vi "getSigProcessing.vi"(0 "Analogue Data (volts)":dbl[][](array[numeric])) -> (1 "Labelled Signals":string[][](array[string]), 2 "Channel Names":string[](array[string]), 3 "Raw Signals":dbl[][](array[numeric]))   [LabVIEW 2013]
uses:
  Globals/measurementGlobal.vi
panel:
  out "Chell Chans.":dbl[](array[numeric])
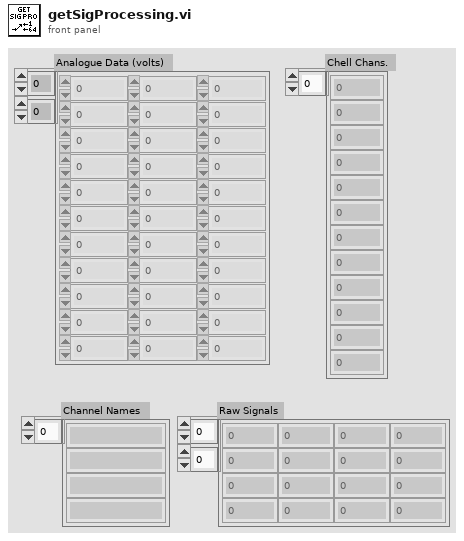
[diagram p1: front panel]
types:
  T1 = typedef "chanType.ctl" = enum16{"Default", "Clock", "Pressure Scanner"}
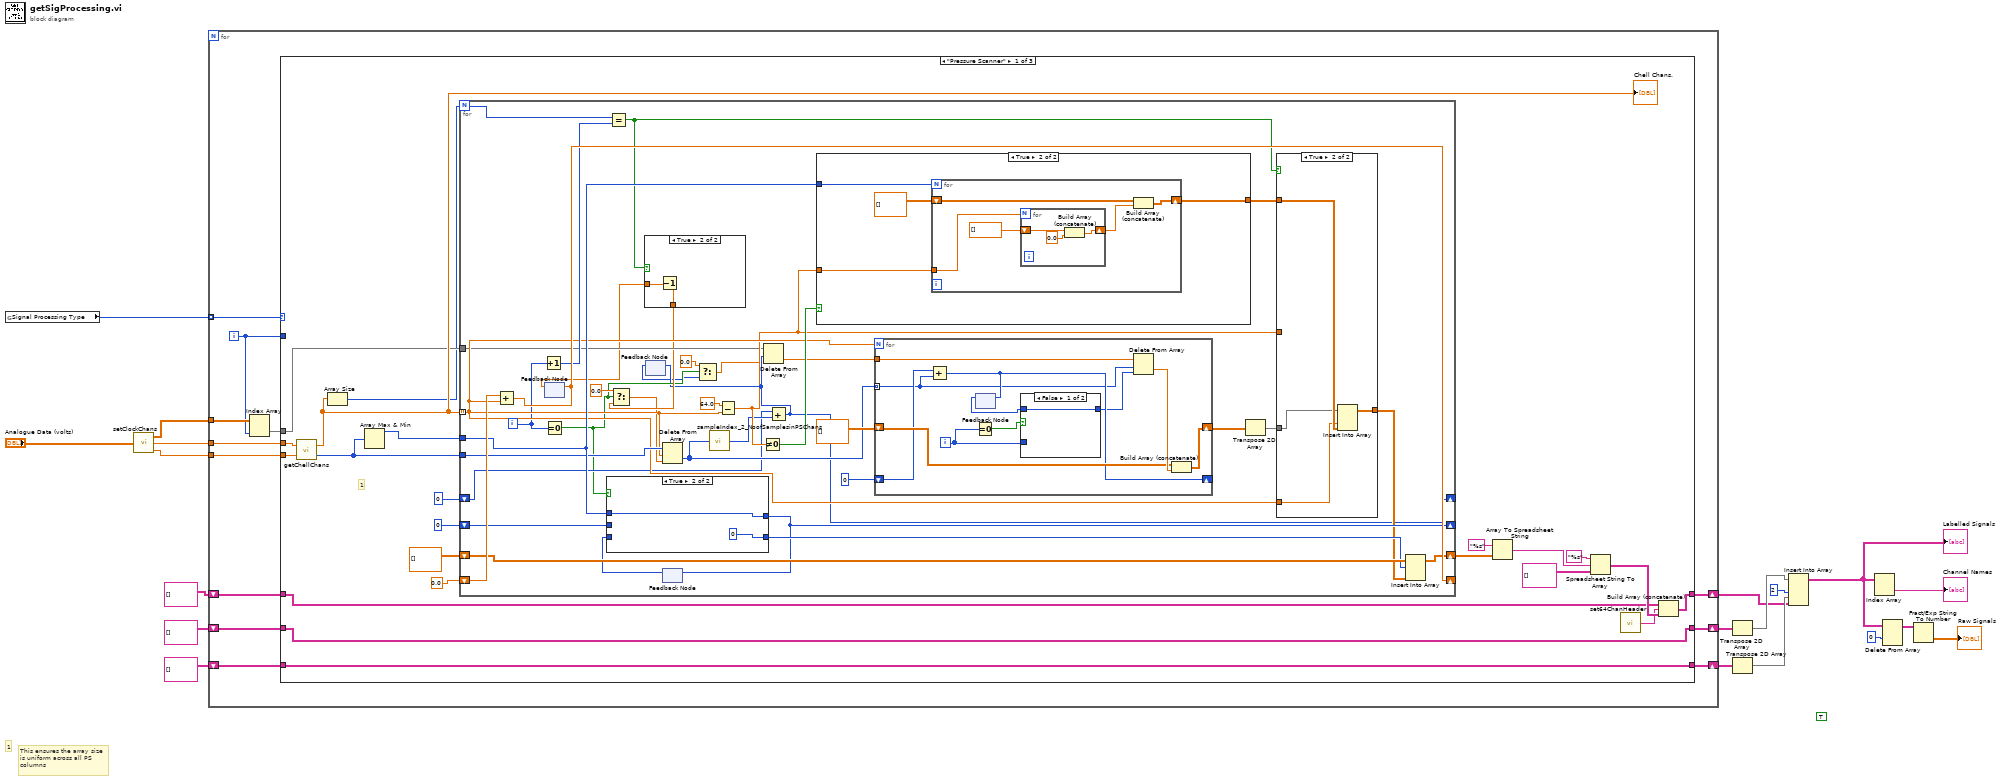
[diagram p0: block diagram]
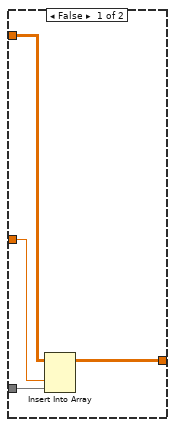
[diagram p3: hidden frame]
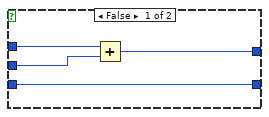
[diagram p4: hidden frame]
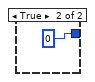
[diagram p5: hidden frame]
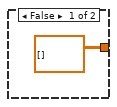
[diagram p6: hidden frame]
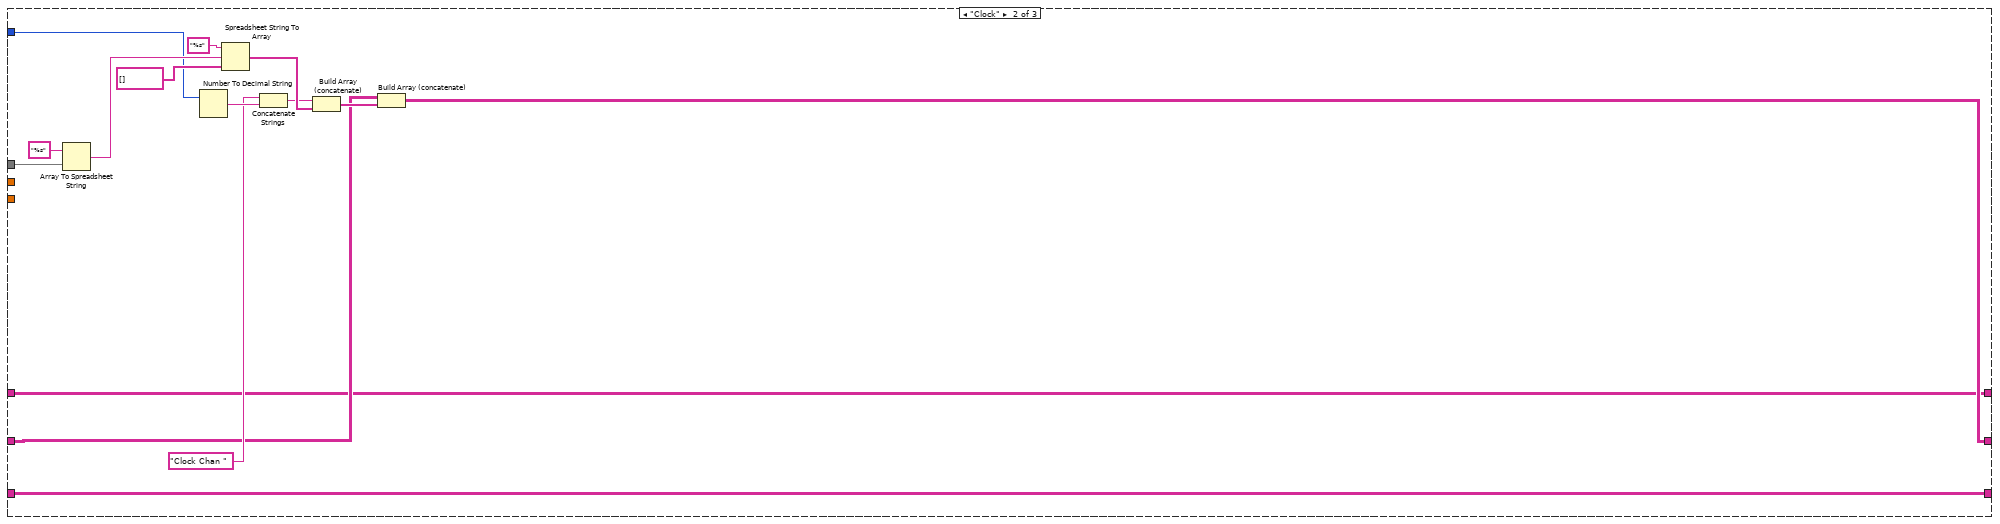
[diagram p7: hidden frame]
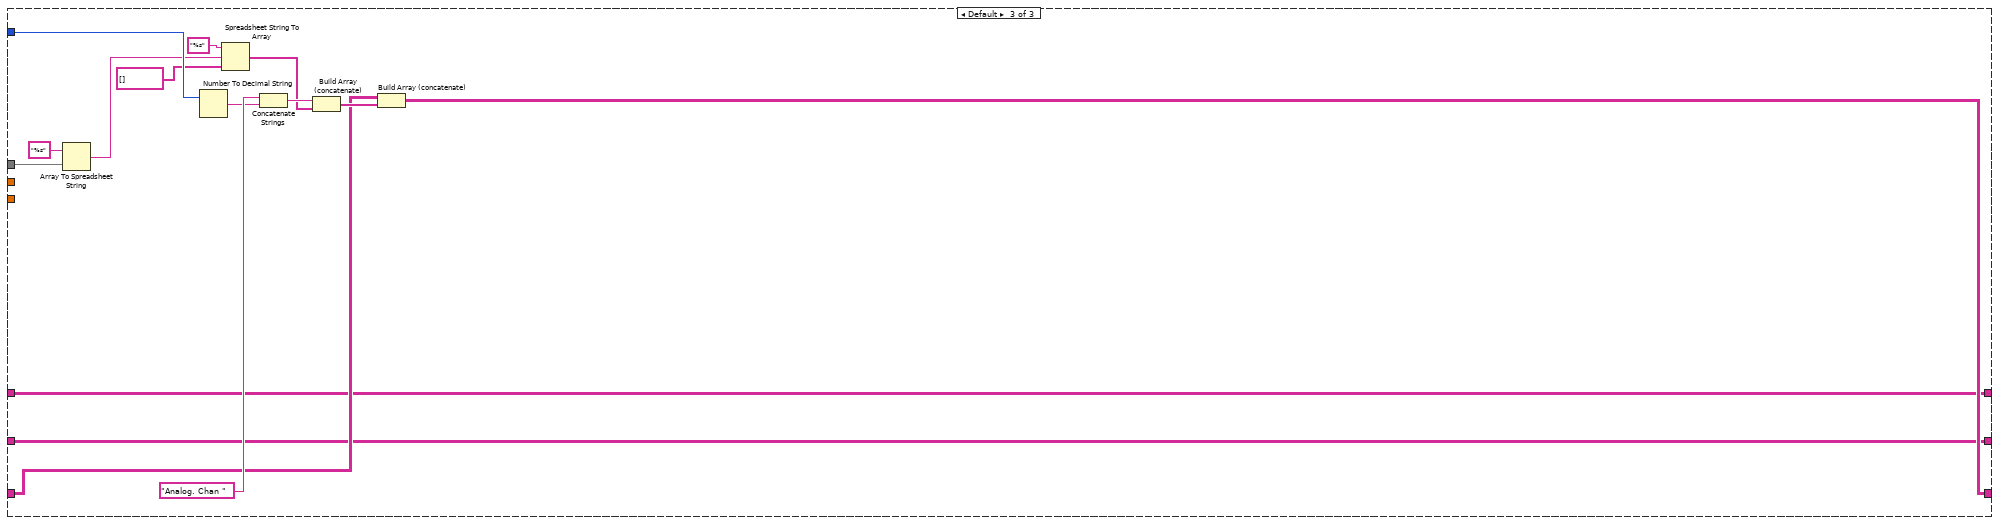
[diagram p8: hidden frame]
diagram:
  (unwired) TRUE
  # "1"
  # "This ensures the array size\nis uniform across all PS\ncolumns"
  n1 = global read "measurementGlobal.vi" "Signal Processing Type"() -> (w19:T1[])
  n2 = call "setClockChans.vi"("Analogue Data (volts)"="Analogue Data (volts)") -> ("Modified Analogue Data (volts)"=w12:dbl[][], "MSB"=w11:dbl[], "LSB"=w10:dbl[])
  n3 = for {
    tunnel: w19 -> [w20] mode=indexing
    tunnel: w12 -> [w30]
    tunnel: w11 -> [w29]
    tunnel: w10 -> [w28]
    shift-right: [w25] -> w7
    shift-left: string[][] [] -> [w26]
    shift-right: [w23] -> w3
    shift-left: string[][] [] -> [w24]
    shift-right: [w21] -> w1
    shift-left: string[][] [] -> [w22]
    i -> [w27]
    n4 = Index Array(array=w30, index (col)=w27) -> (element=w31:dbl[])  [unwired: 1 in]
    n5 = case shown="\"Pressure Scanner\"" w20 {
      tunnel: w31 -> [w45 w140 w150]
      tunnel: w29 -> [w53 _ _]
      tunnel: w28 -> [w52 _ _]
      tunnel: w27 -> [_ w141 w163]
      tunnel: w26 -> [w39 w138 w152]
      tunnel: [w39 w137 w152] -> w25
      tunnel: w24 -> [w38 w136 w154]
      tunnel: [w38 w136 w153] -> w23
      tunnel: w22 -> [w37 w135 w151]
      tunnel: [w36 w135 w151] -> w21
      frame "Pressure Scanner" {
        # "1"
        n6 = call "getChellChans.vi"("LSB"=w52, "MSB"=w53) -> ("Sample Index"=w51:i32[], "No. Chell Chans."=w48:dbl[])
        "Chell Chans." <- w48
        n7 = Array Size(array=w48) -> (size(s)=w33:i32)
        n8 = Array Max & Min(array=w51) -> (max value=w50:i32)  [unwired: 3 out]
        n9 = for {
          N: w33 -> [w77]
          tunnel: w48 -> [w74] mode=indexing
          tunnel: w45 -> [w69]
          tunnel: w51 -> [w79]
          tunnel: w50 -> [w84]
          shift-right: [w87] -> _
          shift-left: 0.0 -> [w88]
          shift-right: [w85] -> w35
          shift-left: dbl[][] [] ("array") -> [w86]
          shift-right: [w81] -> _
          shift-left: 0 -> [w82]
          shift-right: [w56] -> _
          shift-left: 0 -> [w59]
          i -> [w71]
          n10 = Add(x=w88, y=w74) -> (x+y=w87:dbl)
          n11 = Increment(x=w71) -> (x+1=w76:i32)
          n12 = feedback #1() -> (w64:dbl)  [unwired: 1 in]
          n13 = feedback-in #1(w87) -> ()
          n14 = Equal To 0?(x=w71) -> (x = 0?=w58:bool)
          n15 = Equal?(x=w77, y=w76) -> (x = y?=w65:bool)
          n16 = case shown="True" w65 {
            tunnel: w64 -> [w92 w94]
            tunnel: [w92 w93] -> w62
            frame False {
            }
            frame True {
              n17 = Decrement(x=w94) -> (x-1=w93:dbl)
            }
          }
          n18 = Select(t=0.0, s=w58, f=w62) -> (s? t:f=w61:dbl)
          n19 = feedback #2() -> (w55:i32)  [unwired: 1 in]
          n20 = Delete From Array(array=w79, length=w74, index=w61) -> (deleted portion=w66:i32[])  [unwired: 1 out]
          n21 = feedback #3() -> (w80:i32)  [unwired: 1 in]
          n22 = case shown="True" w58 {
            tunnel: w84 -> [w105 w108]
            tunnel: [w103 0] -> w83
            tunnel: w82 -> [w106 _]
            tunnel: [w104 w108] -> w81
            tunnel: w80 -> [w103 _]
            frame False {
              n23 = Add(x=w105, y=w106) -> (x+y=w104:i32)
            }
            frame True {
            }
          }
          n24 = feedback-in #3(w81) -> ()
          n25 = Select(t=0.0, s=w58, f=w55) -> (s? t:f=w54:dbl)
          n26 = call "sampleIndex_2_NoofSamplesinPSChans.vi"("Sample Index"=w66) -> ("No of Samples in PS Chans"=w60:i32)
          n27 = Subtract(x=64.0 ("y"), y=w74) -> (x-y=w73:dbl)
          n28 = Not Equal To 0?(x=w73) -> (x != 0?=w78:bool)
          n29 = Add(x=w59, y=w60) -> (x+y=w56:i32)
          n30 = feedback-in #2(w56) -> ()
          n31 = Delete From Array(array=w69, length=w56, index=w54) -> (deleted portion=w68:dbl[])  [unwired: 1 out]
          n32 = case shown="True" w78 {
            tunnel: w73 -> [_ w123]
            tunnel: [dbl[][] [] w126] -> w75
            tunnel: w84 -> [_ w125]
            frame False {
            }
            frame True {
              n33 = for {
                N: w125 -> [_]
                shift-right: [w128] -> w126
                shift-left: dbl[][] [] -> [w129]
                tunnel: w123 -> [w127]
                n34 = for {
                  N: w127 -> [_]
                  shift-right: [w133] -> w130
                  shift-left: dbl[] [] -> [w134]
                  n35 = Build Array (concatenate)(w134, 0.0) -> (w133:dbl[])
                }
                n36 = Build Array (concatenate)(w129, w130) -> (w128:dbl[][])
              }
            }
          }
          n37 = for {
            N: w74 -> [_]
            tunnel: w66 -> [w112] mode=indexing
            tunnel: w68 -> [w119]
            shift-right: [w117] -> w70
            shift-left: dbl[][] [] ("element") -> [w116]
            shift-right: [w114] -> _
            shift-left: 0 -> [w115]
            i -> [w111]
            n38 = Add(x=w115, y=w112) -> (x+y=w114:i32)
            n39 = feedback-in #4(w114) -> ()
            n40 = feedback #4() -> (w113:i32)  [unwired: 1 in]
            n41 = Equal To 0?(x=w111) -> (x = 0?=w110:bool)
            n42 = case shown="False" w110 {
              tunnel: [w120 0] -> w109
              tunnel: w111 -> [_ _]
              tunnel: w113 -> [w120 _]
              frame False {
              }
              frame True {
              }
            }
            n43 = Delete From Array(array=w119, length=w112, index=w109) -> (deleted portion=w118:dbl[])  [unwired: 1 out]
            n44 = Build Array (concatenate)(w116, w118) -> (w117:dbl[][])
          }
          n45 = Transpose 2D Array(2D array=w70) -> (transposed array=w67:dbl[][])
          n46 = case shown="True" w65 {
            tunnel: w75 -> [w98 w102]
            tunnel: w67 -> [w97 w101]
            tunnel: w74 -> [_ w99]
            tunnel: w73 -> [w96 _]
            tunnel: [w95 w100] -> w72
            frame False {
              n47 = Insert Into Array(array=w98, index (col)=w96, new element=w97) -> (w95:dbl[][])  [unwired: 1 in]
            }
            frame True {
              n48 = Insert Into Array(array=w101, index (col)=w99, new element=w102) -> (w100:dbl[][])  [unwired: 1 in]
            }
          }
          n49 = Insert Into Array(array=w86, index (row)=w83, new element=w72) -> (w85:dbl[][])  [unwired: 1 in]
        }
        n50 = Array To Spreadsheet String(array=w35, 3:"%s" ("format string")) -> (spreadsheet string=w43:string)  [unwired: 1 in]
        n51 = Spreadsheet String To Array(format string="%s", spreadsheet string=w43, array type (2D Dbl)=string[][] []) -> (array=w40:string[][])  [unwired: 1 in]
        n52 = call "set64ChanHeader.vi"() -> ("64 Chan Header"=w34:string[])
        n53 = Build Array (concatenate)(w37, w34, w40) -> (w36:string[][])
      }
      frame "Clock" {
        n54 = Array To Spreadsheet String(array=w140, 3:"%s" ("format string")) -> (spreadsheet string=w145:string)  [unwired: 1 in]
        n55 = Number To Decimal String(number=w141) -> (decimal integer string=w143:string)  [unwired: 1 in]
        n56 = Spreadsheet String To Array(format string="%s", spreadsheet string=w145, array type (2D Dbl)=string[] []) -> (array=w149:string[])  [unwired: 1 in]
        n57 = Concatenate Strings("Clock Chan " ("string"), w143) -> (w148:string)
        n58 = Build Array (concatenate)(w148, w149) -> (w139:string[])
        n59 = Build Array (concatenate)(w138, w139) -> (w137:string[][])
      }
      frame Default {
        n60 = Array To Spreadsheet String(array=w150, 3:"%s" ("format string")) -> (spreadsheet string=w160:string)  [unwired: 1 in]
        n61 = Number To Decimal String(number=w163) -> (decimal integer string=w162:string)  [unwired: 1 in]
        n62 = Spreadsheet String To Array(format string="%s", spreadsheet string=w160, array type (2D Dbl)=string[] []) -> (array=w156:string[])  [unwired: 1 in]
        n63 = Concatenate Strings("Analog. Chan " ("string"), w162) -> (w157:string)
        n64 = Build Array (concatenate)(w157, w156) -> (w155:string[])
        n65 = Build Array (concatenate)(w154, w155) -> (w153:string[][])
      }
    }
  }
  n66 = Transpose 2D Array(2D array=w7) -> (transposed array=w5:string[][])
  n67 = Transpose 2D Array(2D array=w3) -> (transposed array=w2:string[][])
  n68 = Insert Into Array(array=w5, index (col)=2 ("disabled index (col)"), new element #1=w2, new element #2=w1) -> (w14:string[][])  [unwired: 1 in]
  "Labelled Signals" <- w14
  n69 = Index Array(array=w14) -> (element=→"Channel Names":string[])  [unwired: 2 in]
  n70 = Delete From Array(array=w14, index (row)=0) -> (array with subset deleted=w16:string[][])  [unwired: 2 in, 1 out]
  n71 = Fract/Exp String To Number(string=w16) -> (number=→"Raw Signals":dbl[][])  [unwired: 3 in, 1 out]
